vi "AddToOldMasters.vi"(3 "Address":string) -> ()   [LabVIEW 2018]
doc: "Adds an IP address to the list of Masters"
uses:
  <userlib>/ROS for LabVIEW Software/ROS/Code/_ROSDefinition.vi
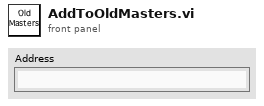
[diagram p1: front panel]
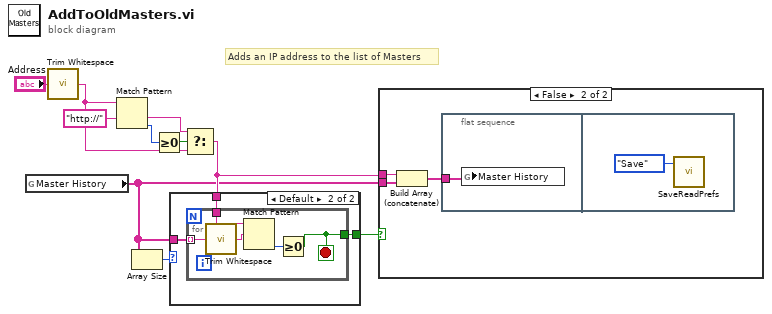
[diagram p0: block diagram]
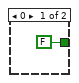
[diagram p2: hidden frame]
diagram:
  # "Adds an IP address to the list of Masters"
  n1 = global read "_ROSDefinition.vi" "Master History"() -> (w1:string[])
  n2 = call <vilib>:"Trim Whitespace.vi"("string"="Address") -> ("trimmed string"=w5:string)  [unwired: 1 in]
  n3 = Match Pattern(string=w5, regular expression="http://") -> (after substring=w7:string, offset past match=w9:i32)  [unwired: 1 in, 2 out]
  n4 = Array Size(array=w1) -> (size(s)=w2:i32)
  n5 = Greater Or Equal To 0?(x=w9) -> (x >= 0?=w8:bool)
  n6 = Select(t=w7, s=w8, f=w5) -> (s? t:f=w4:string)
  n7 = case shown="Default" w2 {
    tunnel: w4 -> [_ w14]
    tunnel: w1 -> [_ w13]
    tunnel: [FALSE w12] -> w3
    frame 0 {
    }
    frame Default {
      n8 = for {
        tunnel: w14 -> [w19]
        tunnel: w13 -> [w18] mode=indexing
        tunnel: [w15] -> w12
        stop <- w15 stop-if-true
        n9 = call <vilib>:"Trim Whitespace.vi"("string"=w18) -> ("trimmed string"=w17:string)  [unwired: 1 in]
        n10 = Match Pattern(string=w19, regular expression=w17) -> (offset past match=w16:i32)  [unwired: 1 in, 3 out]
        n11 = Greater Or Equal To 0?(x=w16) -> (x >= 0?=w15:bool)
      }
    }
  }
  n12 = case shown="False" w3 {
    tunnel: w1 -> [_ w22]
    tunnel: w4 -> [_ w21]
    frame True {
    }
    frame False {
      n13 = Build Array (concatenate)(w21, w22) -> (w20:string[])
      n14 = flat-sequence {
        tunnel: w20 -> [w23]
        frame #0 {
          n15 = global write "_ROSDefinition.vi" "Master History"(w23) -> ()
        }
        frame #1 {
          n16 = call <userlib>:"SaveReadPrefs.vi"("Task"=enum16{"Read", "Save"}."Save") -> ()  [unwired: 2 in, 1 out]
        }
      }
    }
  }
